vi "SetFreqCentSpan.vi"(0 "VISA IN":refnum<visa-resource-name>, 3 "Center Frequency":dbl=10000000.0, 4 "Span":dbl=10000000.0, 5 "error in":errorcluster, 6 "Channel":i32=1) -> (14 "VISA Out":refnum<visa-resource-name>, 19 "error out":errorcluster)   [LabVIEW 2018, in "PNA-X.lvlib"]
uses:
  PNA-X.lvlib
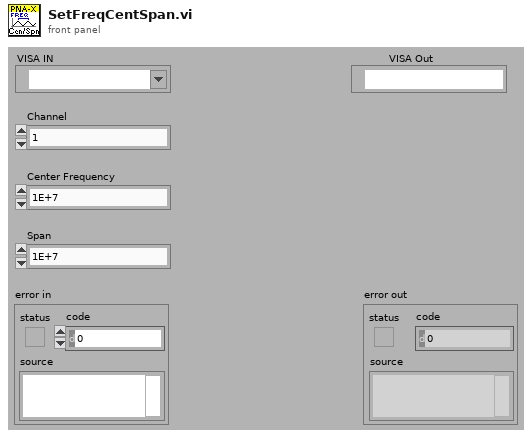
[diagram p1: front panel]
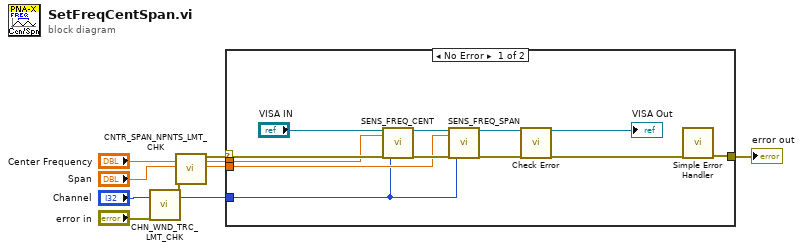
[diagram p0: block diagram]
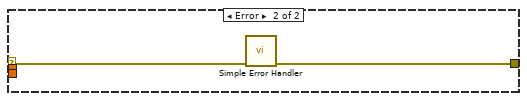
[diagram p2: hidden frame]
diagram:
  n1 = call "CHN_WND_TRC_LMT_CHK.vi"("Channel"="Channel", "error in"="error in") -> ("error out"=w5:errorcluster, "Channel"=w3:i32)  [unwired: 13 in, 3 out]
  n2 = call "CNTR_SPAN_NPNTS_LMT_CHK.vi"("Center"="Center Frequency", "Span"="Span", "error in"=w5) -> ("error out"=w9:errorcluster, "Center"=w8:dbl, "Span"=w7:dbl)  [unwired: 13 in, 1 out]
  n3 = case shown="No Error" w9 {
    selector: w9 -> [w22 w24]
    tunnel: [w18 w23] -> w10
    tunnel: w8 -> [w13 _]
    tunnel: w7 -> [w12 _]
    tunnel: w3 -> [w11 _]
    frame No Error {
      n4 = call "SENS_FREQ_CENT.vi"("VISA IN"="VISA IN", "Center Frq."=w13, "error in"=w22, "Channel"=w11) -> ("VISA Out"=w16:refnum<visa-resource-name>, "error out"=w21:errorcluster)  [unwired: 14 in]
      n5 = call "SENS_FREQ_SPAN.vi"("VISA IN"=w16, "Frq. Span"=w12, "error in"=w21, "Channel"=w11) -> ("VISA Out"=w15:refnum<visa-resource-name>, "error out"=w20:errorcluster)  [unwired: 14 in]
      n6 = call "Check Error.vi"("VISA Resource Name"=w15, "error in (no error)"=w20) -> ("dup VISA session"=→"VISA Out":refnum<visa-resource-name>, "error out"=w19:errorcluster)  [unwired: 16 in]
      n7 = call <vilib>:"Simple Error Handler.vi"("error in (no error)"=w19) -> ("error out"=w18:errorcluster)  [unwired: 4 in, 4 out]
    }
    frame Error {
      n8 = call <vilib>:"Simple Error Handler.vi"("error in (no error)"=w24) -> ("error out"=w23:errorcluster)  [unwired: 4 in, 4 out]
    }
  }
  "error out" <- w10
